vi "To bytes.vi"(3 "MsgPackTimestamp in":refnum<class "MsgPackTimestamp.lvclass">) -> (1 "Array":u8[](array[numeric]))   [LabVIEW 2020, in "MessagePack.lvlib" / "MsgPackTimestamp.lvclass"]
uses:
  MsgPackTimestamp.lvclass
  MsgPackTimestamp.lvclass/MsgPackTimestamp.ctl
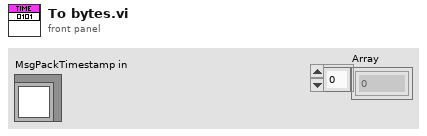
[diagram p1: front panel]
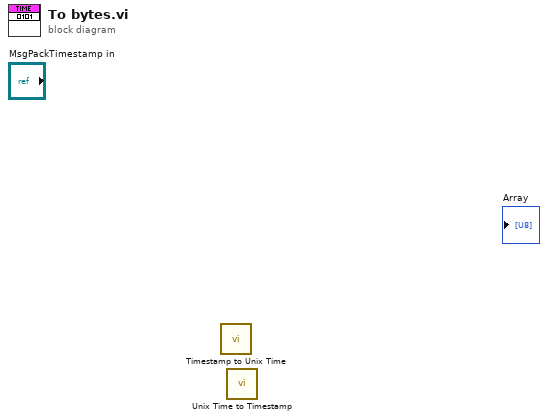
[diagram p0: block diagram]
diagram:
  n1 = call <vilib>:"Timestamp to Unix Time.vi"() -> ()  [unwired: 10 in, 2 out]
  n2 = call <vilib>:"Unix Time to Timestamp.vi"() -> ()  [unwired: 10 in, 2 out]
